vi "control_queues_obtain.vi"(6 "error in":errorcluster, 8 "Process names in":string[](array[string])=["DAQ", "pixel_mapper", "averager", "display", "pockels", "storage"], 9 "Process_communication in":variant) -> (0 "error out":errorcluster, 3 "Process_communication out":variant)   [LabVIEW 2011, in "Fiberscope_library.lvlib"]
uses:
  Fiberscope_library.lvlib
  typedefs/control_process_state_cluster.ctl
  typedefs/control_process_state_enum.ctl
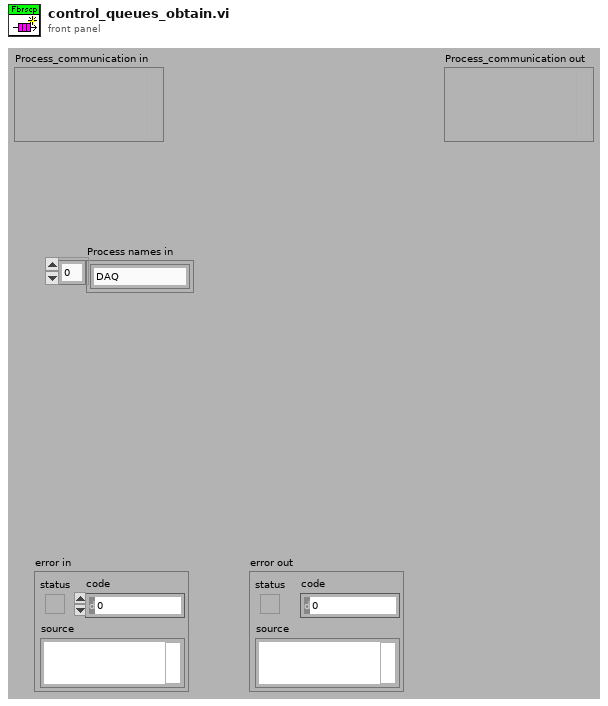
[diagram p1: front panel]
types:
  T1 = typedef "Fiberscope_library.lvlib/control_process_state_cluster.ctl" = cluster{"Control_process_state_enum":T2, "variant":variant}
  T2 = typedef "Fiberscope_library.lvlib/control_process_state_enum.ctl" = enum16{"Init", "Quit", "Start", "Stop", "Change_parameters", "Running", "Finish", "Custom"}
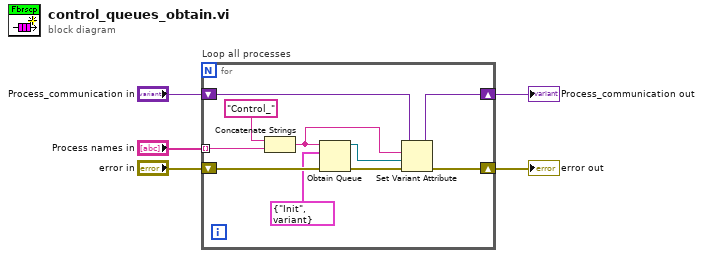
[diagram p0: block diagram]
diagram:
  n1 = for "Loop all processes" {
    tunnel: "Process names in" -> [w7] mode=indexing
    shift-right: [w11] -> w4
    shift-left: "error in" -> [w15]
    shift-right: [w8] -> w1
    shift-left: "Process_communication in" -> [w9]
    n2 = Concatenate Strings("Control_" ("string"), w7) -> (w6:string)
    n3 = Obtain Queue(name (unnamed)=w6, element data type=T1 {"Control_process_state_enum"=enum."Init", "variant"=variant} ("Control_process_state_cluster"), error in (no error)=w15) -> (queue out=w10:refnum<queue>, error out=w12:errorcluster)  [unwired: 2 in, 1 out]
    n4 = Set Variant Attribute(Variant=w9, name=w6, value=w10, error in=w12) -> (Variant out=w8:variant, error out=w11:errorcluster)  [unwired: 1 out]
  }
  "error out" <- w4
  "Process_communication out" <- w1
